vi "Set Motor Voltage.vi"(11 "Reference Voltage in":dbl) -> (3 "Reference Voltage out":dbl)   [LabVIEW 2018]
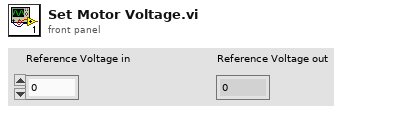
[diagram p1: front panel]
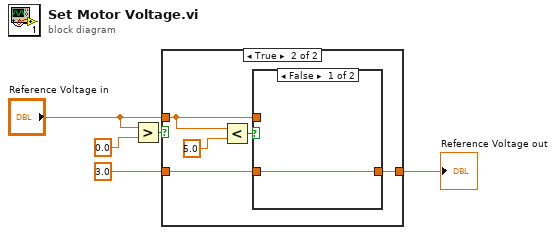
[diagram p0: block diagram]
diagram:
  n1 = Greater?(x="Reference Voltage in", y=0.0) -> (0:w1:bool)
  n2 = case shown="True" w1 {
    tunnel: "Reference Voltage in" -> [_ w9]
    tunnel: [w6 w8] -> w4
    tunnel: 3.0 -> [w6 w7]
    frame False {
    }
    frame True {
      n3 = Less?(x=w9, y=5.0) -> (x < y?=w11:bool)
      n4 = case shown="False" w11 {
        tunnel: w9 -> [_ w13]
        tunnel: [w12 w13] -> w8
        tunnel: w7 -> [w12 _]
        frame False {
        }
        frame True {
        }
      }
    }
  }
  "Reference Voltage out" <- w4
